vi "Latch.vi"(10 "Reset":bool, 11 "Input":bool) -> (3 "Output":bool)   [LabVIEW 2017]
doc: "When input goes true the output stays true forever"
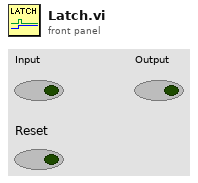
[diagram p1: front panel]
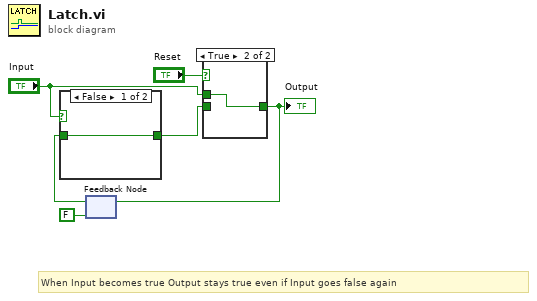
[diagram p0: block diagram]
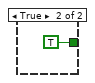
[diagram p3: hidden frame]
diagram:
  # "When Input becomes true Output stays true even if Input goes false again"
  n1 = feedback #1(FALSE ("Output")) -> (w6:bool)
  n2 = case shown="False" "Input" {
    tunnel: [w7 TRUE ("Output")] -> w1
    tunnel: w6 -> [w7 _]
    frame False {
    }
    frame True {
    }
  }
  n3 = case shown="True" "Reset" {
    tunnel: [w9 w10] -> w3
    tunnel: "Input" -> [_ w10]
    tunnel: w1 -> [w9 _]
    frame False {
    }
    frame True {
    }
  }
  "Output" <- w3
  n4 = feedback-in #1(w3) -> ()
